vi "Load Report 2.vi"(8 "error in (no error)":errorcluster, 11 "HIJ Vision File Display In":refnum<class "HIJ Vision File Display.lvclass">) -> (0 "error out":errorcluster, 3 "HIJ Vision File Display Out":refnum<class "HIJ Vision File Display.lvclass">)   [LabVIEW 2014, in "HIJ Vision File Display.lvlib" / "HIJ Vision File Display.lvclass"]
uses:
  HIJ Vision File Display.lvclass
  HIJ Vision File Display.lvclass/HIJ Vision File Display.ctl
  HIJ Vision Display/HIJ Vision Display/HIJ Vision Display.lvclass/HIJ Vision Display.ctl
  Analyze/Analyze Actor/Analyze Actor Messages/Load Parameters Msg/Load Parameters Msg.lvclass/Load Parameters Msg.ctl
  <vilib>/ActorFramework/Message Enqueuer/Message Enqueuer.lvclass/Message Enqueuer.ctl
  HIJ Vision Display/HIJ Vision Display/Read Analyze Actor.vi
  <vilib>/ActorFramework/Message Enqueuer/Enqueue.vi
  <vilib>/ActorFramework/Message Priority Queue/Priority Enqueue.vi
  <vilib>/ActorFramework/Message Enqueuer/Message Enqueuer.lvclass
  Analyze/Analyze Actor/Analyze Actor Messages/Load Parameters Msg/Load Parameters Msg.lvclass
  HIJ Vision Display/HIJ Vision Display/HIJ Vision Display.lvclass
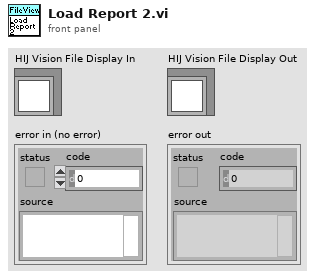
[diagram p1: front panel]
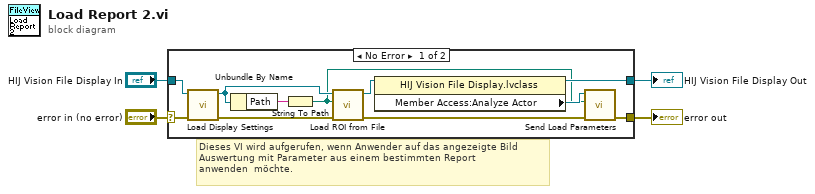
[diagram p0: block diagram]
diagram:
  # "Dieses VI wird aufgerufen, wenn Anwender auf das angezeigte Bild\nAuswertung mit Parameter aus einem bestimmten Report \nanwenden  möchte."
  n1 = case shown="No Error" "error in (no error)" {
    selector: "error in (no error)" -> [w10 w17]
    tunnel: [w14 w17] -> w3
    tunnel: [w7 w16] -> w1
    tunnel: "HIJ Vision File Display In" -> [w15 w16]
    frame No Error {
      n2 = call-dynamic "Load Display Settings.vi"("error in (no error)"=w10, "AF IMAQ Display in"=w15) -> ("error out"=w12:errorcluster, "AF IMAQ Display out"=w9:refnum<class "HIJ Vision File Display.lvclass">)  [unwired: 8 in]
      n3 = Unbundle By Name(w9) -> ("Path"=w8:string)
      n4 = String To Path(string=w8) -> (path=w5:path)
      n5 = call "Load ROI from File.vi"("error in (no error)"=w12, "Report File"=w5, "IMAQ Display in"=w9) -> ("error out"=w11:errorcluster, "IMAQ Display out"=w13:refnum<class "HIJ Vision File Display.lvclass">)  [unwired: 7 in]
      n6 = property class="HIJ Vision File Display.lvclass"(reference=w13) -> (reference out=w7:refnum<class "HIJ Vision File Display.lvclass">, "Member Access:Analyze Actor"=w6:refnum<class "Message Enqueuer.lvclass">)  [unwired: 1 in, 1 out]
      n7 = call "Send Load Parameters.vi"("error in (no error)"=w11, "Resource"=w5, "Message Enqueuer"=w6) -> ("error out"=w14:errorcluster)  [unwired: 7 in, 1 out]
    }
    frame Error {
    }
  }
  "error out" <- w3
  "HIJ Vision File Display Out" <- w1
